vi "Ethernet TCP Update & Write.vi"(1 "Client Info":T1[](array[typedef]), 4 "Minor Frame Freq":u8 caption="Minor Frame Time", 6 "Dynamic Frame Info":T2, 7 "Next Index":i32[][](array[numeric]), 8 "error in":errorcluster, 9 "Interupt Q":refnum<queue>, 10 "Frame Info Array":T3[](array[typedef]), 11 "Connection ID":refnum<k5>[](array[refnum])) -> (0 "error out":errorcluster, 2 "Frame Info Array":T3[](array[typedef]), 3 "Stop":bool, 5 "Next Index":i32[][](array[numeric]))   [LabVIEW 2024]
doc: "All Rights Reserved © 2017 SyncSols"
uses:
  Controls/Ethernet Frame Info Cluster.ctl
  Controls/Ethernet Message Info Cluster.ctl
  Controls/Ethernet Dynamic Data Cluster.ctl
  TCP Engine/Controls/TCP Engine Serial Interupt Cluster.ctl
  Controls/Ethernet Dynamic Frame Info.ctl
  Controls/Ethernet Client Info Cluster.ctl
  TCP Engine/TCP Engine.lvlib
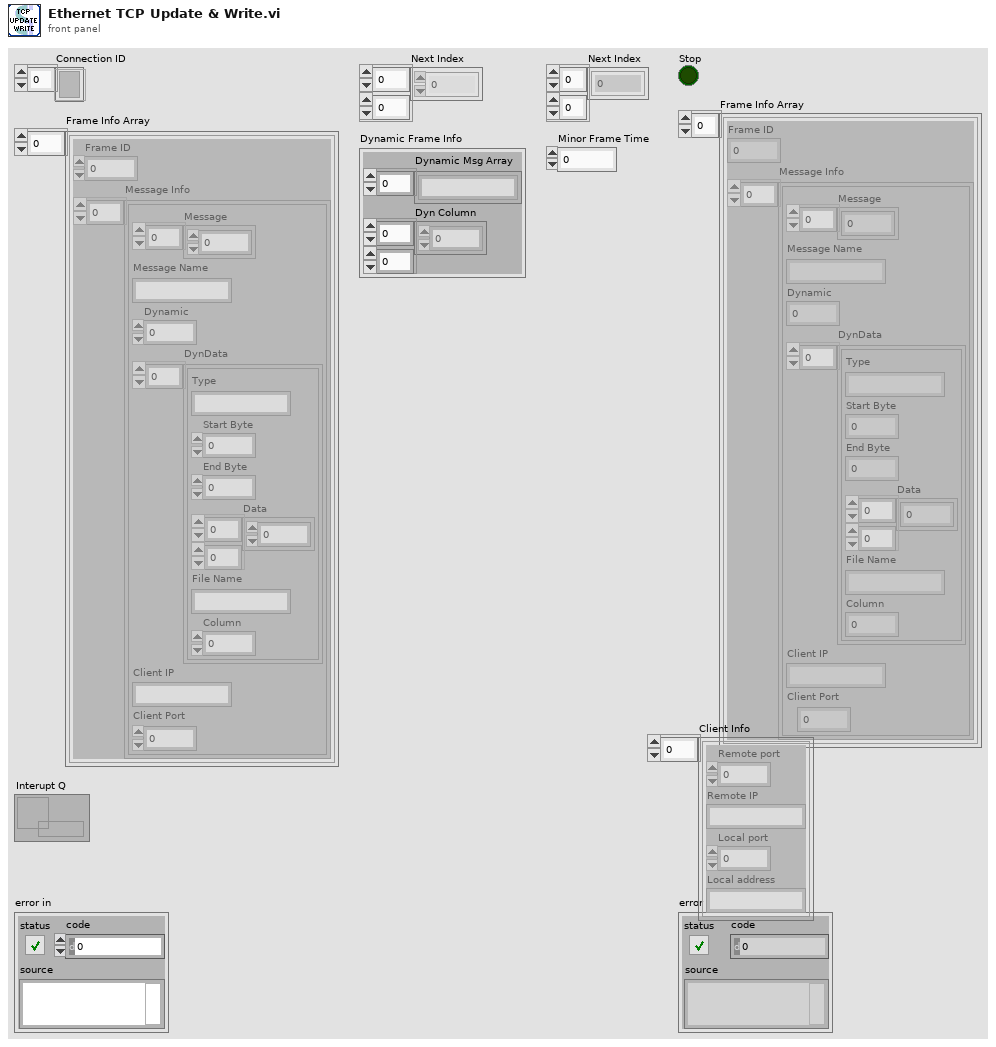
[diagram p1: front panel]
types:
  T1 = typedef "Ethernet Client Info Cluster.ctl" = cluster{"Remote port":u16, "Remote IP":string, "Local port":u16, "Local address":string}
  T2 = typedef "Ethernet Dynamic Frame Info.ctl" = cluster{"Dynamic Msg Array":string[], "Dyn Column":i32[][]}
  T3 = typedef "Ethernet Frame Info Cluster.ctl" = cluster{"Frame ID":u16, "Message Info":T4[]}
  T4 = typedef "Ethernet Message Info Cluster.ctl" = cluster{"Message":u8[], "Message Name":string, "Dynamic":u8, "DynData":T5[], "Client IP":string, "Client Port":u16}
  T5 = typedef "Ethernet Dynamic Data Cluster.ctl" = cluster{"Type":string, "Start Byte":u8, "End Byte":u8, "Data":u32[][], "File Name":string, "Column":i32}
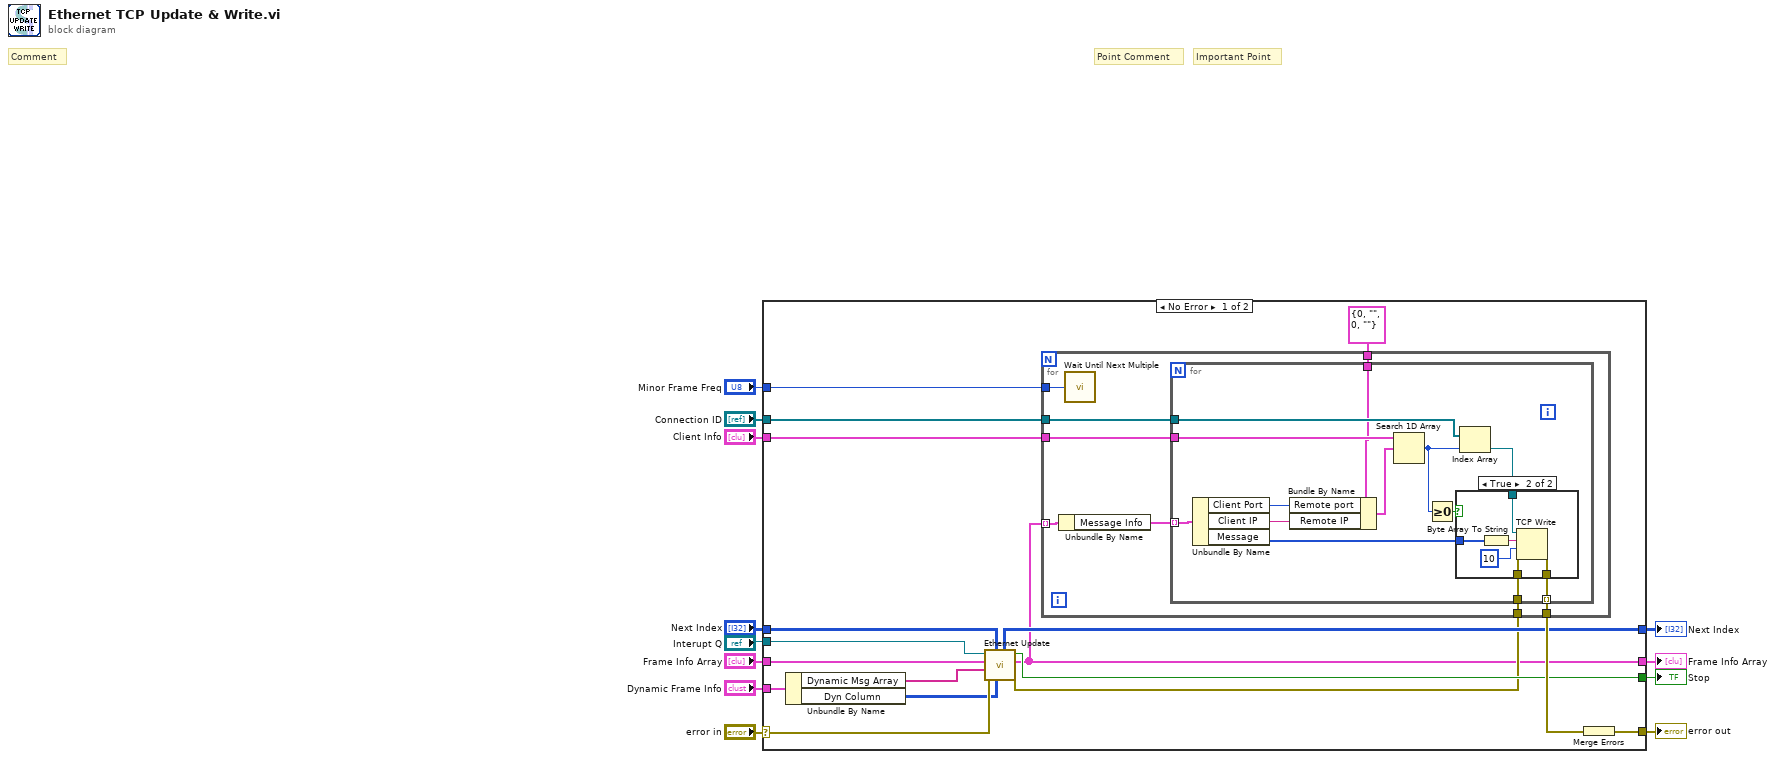
[diagram p0: block diagram]
diagram:
  # "Important Point"
  # "Point Comment"
  # "Comment"
  n1 = case shown="No Error" "error in" {
    selector: "error in" -> [w25 w60]
    tunnel: [w28 w60] -> w10
    tunnel: "Minor Frame Freq" -> [w29 _]
    tunnel: [w16 w59] -> w9
    tunnel: [w23 _] -> w8
    tunnel: "Next Index" -> [w26 w58]
    tunnel: "Frame Info Array" -> [w21 w59]
    tunnel: "Interupt Q" -> [w24 _]
    tunnel: [w22 w58] -> w4
    tunnel: "Dynamic Frame Info" -> [w20 _]
    tunnel: "Client Info" -> [w15 _]
    tunnel: "Connection ID" -> [w14 _]
    frame No Error {
      n2 = Unbundle By Name(w20) -> ("Dynamic Msg Array"=w19:string[], "Dyn Column"=w18:i32[][])
      n3 = call "Ethernet Update.vi"("Dynamic Column"=w18, "Next Index"=w26, "error in"=w25, "Dynamic Msg Array"=w19, "Frame Info Array"=w21, "Interupt Q"=w24) -> ("error out"=w17:errorcluster, "Frame Info Array"=w16:T3[], "Stop"=w23:bool, "Next Index"=w22:i32[][])  [unwired: 2 in]
      n4 = for {
        tunnel: w29 -> [w37]
        tunnel: [w36] -> w27
        tunnel: w17 -> [w34]
        tunnel: w16 -> [w33] mode=indexing
        tunnel: w15 -> [w32]
        tunnel: w14 -> [w31]
        tunnel: T1 {"Remote port"=0, "Remote IP"="", "Local port"=0, "Local address"=""} -> [w30]
        n5 = Unbundle By Name(w33) -> ("Message Info"=w35:T4[])
        n6 = call "Wait Until Next Multiple"("Count(mSec)"=w37) -> ()  [unwired: 1 out]
        n7 = for {
          tunnel: w35 -> [w50] mode=indexing
          tunnel: w34 -> [w48]
          tunnel: [w47] -> w36 mode=indexing
          tunnel: w32 -> [w44]
          tunnel: w31 -> [w42]
          tunnel: w30 -> [w38]
          n8 = Unbundle By Name(w50) -> ("Client Port"=w46:u16, "Client IP"=w45:string, "Message"=w49:u8[])
          n9 = Bundle By Name(cluster=w38, "Remote port"=w46, "Remote IP"=w45) -> (w43:T1)
          n10 = Search 1D Array(1D array=w44, element=w43) -> (index of element=w40:i32)  [unwired: 1 in]
          n11 = Greater Or Equal To 0?(x=w40) -> (x >= 0?=w39:bool)
          n12 = Index Array(array=w42, index=w40) -> (element=w41:refnum<k5>)
          n13 = case shown="True" w39 {
            tunnel: w49 -> [_ w57]
            tunnel: w48 -> [w51 w55]
            tunnel: [w51 w54] -> w47
            tunnel: w41 -> [_ w53]
            frame False {
            }
            frame True {
              n14 = Byte Array To String(unsigned byte array=w57) -> (string=w56:string)
              n15 = TCP Write(connection ID=w53, data in=w56, error in (no error)=w55, 9:10 ("timeout ms (25000)")) -> (error out=w54:errorcluster)  [unwired: 2 out]
            }
          }
        }
      }
      n16 = Merge Errors(w27) -> (w28:errorcluster)
    }
    frame Error {
    }
  }
  "error out" <- w10
  "Stop" <- w8
  "Frame Info Array" <- w9
  "Next Index" <- w4
